vi "Launch Contestant Actors.vi"(8 "error in (no error)":errorcluster, 10 "Contestant Names":string[](array[string]), 11 "Controller in":refnum<class "Controller.lvclass">) -> (0 "error out":errorcluster, 3 "Controller out":refnum<class "Controller.lvclass">)   [LabVIEW 2024, in "Controller.lvlib" / "Controller.lvclass"]
uses:
  Controller.lvclass
  Controller.lvclass/Controller.ctl
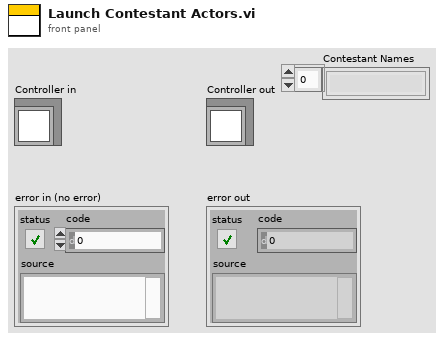
[diagram p1: front panel]
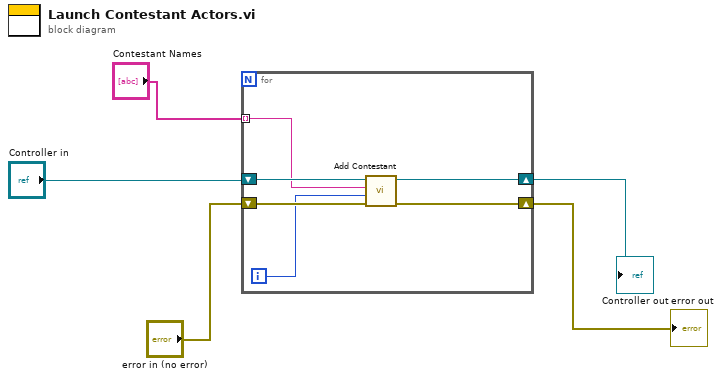
[diagram p0: block diagram]
diagram:
  n1 = for {
    shift-right: [w9] -> w4
    shift-left: "Controller in" -> [w11]
    shift-right: [w8] -> w3
    shift-left: "error in (no error)" -> [w10]
    tunnel: "Contestant Names" -> [w6] mode=indexing
    i -> [w7]
    n2 = call-dynamic "Add Contestant.vi"("error in (no error)"=w10, "Position"=w7, "Name"=w6, "Controller in"=w11) -> ("error out"=w8:errorcluster, "Controller out"=w9:refnum<class "Controller.lvclass">)  [unwired: 6 in]
  }
  "Controller out" <- w4
  "error out" <- w3
